vi "beginOneTouchShot.vi"(4 "Gap Coord":dbl[](array[numeric]), 6 "bestY":dbl, 8 "error in (no error)":errorcluster, 9 "Robot":refnum<class "Robot.lvclass">, 10 "Game":refnum<class "Game.lvclass">, 11 "ShootTactic in":refnum<class "ShootTactic.lvclass">) -> (0 "error out":errorcluster, 2 "Boolean":bool, 3 "ShootTactic out":refnum<class "ShootTactic.lvclass">)   [LabVIEW 2023]
uses:
  ShootTactic.lvclass
  Game_class/Game.lvclass
  Robot_class/Robot.lvclass
  Game_class/Game.lvclass/Game.ctl
  Robot_class/Robot.lvclass/Robot.ctl
  Parameters_class/Parameters.lvclass/Parameters.ctl
  Parameters_class/Read AttakingOurselves.vi
  Robot_class/Read role.vi
  Robot_class/Read Zone.vi
  Game_class/Read Parameters.lvclass.vi
  Game_class/Read BallRef.vi
  Game_class/Read KeeperTeam.vi
  Game_class/Read NewParameters.vi
  Game_class/Read FieldRef.vi
  Parameters_class/Parameters.lvclass
  Ball_class/Ball.lvclass
  Ally_class/Ally.lvclass
  Utilities_class/Style.ctl
  Field_class/Field.lvclass
  Zone_class/Zone.lvclass
  Team_class/KeeperPlay.ctl
  Utilities_class/Utilities.lvclass
panel:
  out "Evaluation":dbl
  out "appended array":bool[](array[boolean])
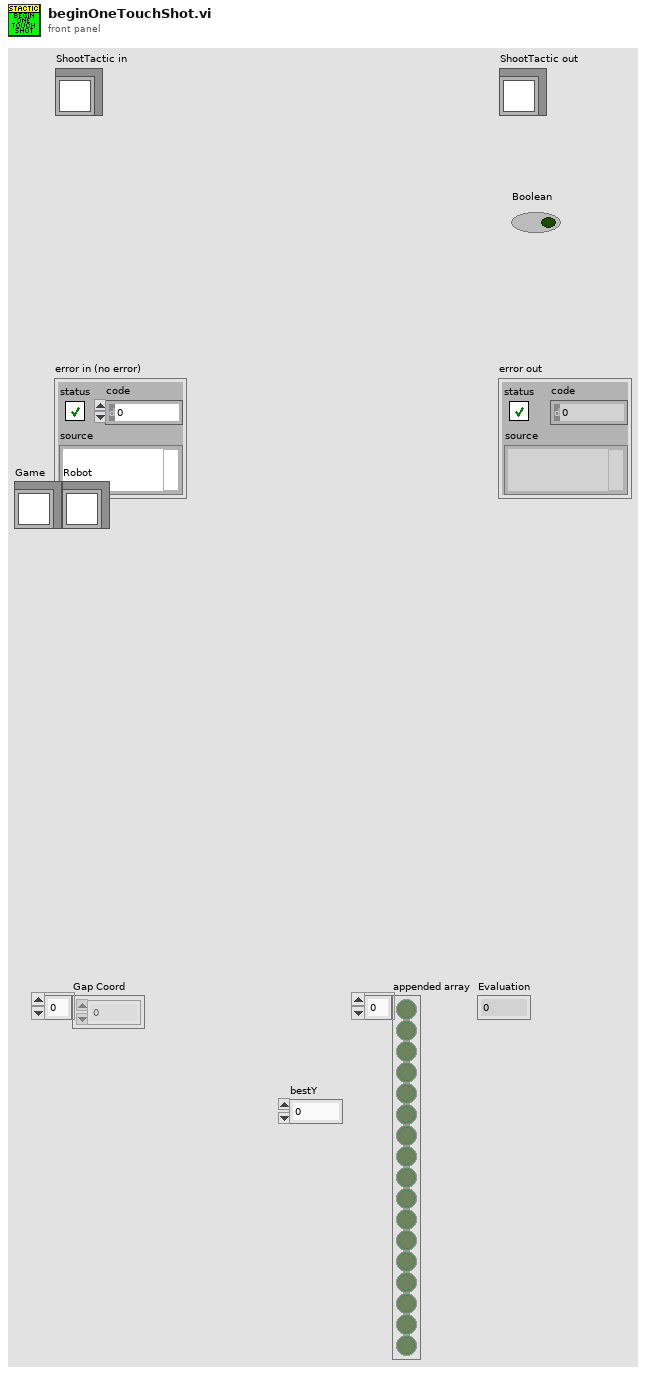
[diagram p1: front panel]
types:
  T1 = typedef "NewParameters.ctl" = cluster{"PenaltyDistance":dbl, "DistanceAttackerToBackBall":dbl, "Division":enum16{"Div B", "Div A"}, "DistanceToAvoidyEnemyRobot":dbl, "BallPlacementDistance":dbl, "DisatanceBehindBallToStealBall":dbl, "MaxDistanceToPositionKickoff":dbl, "BlockEnemyTarget":bool, "MaxStopVAng":dbl, "DistanceMarkerToEnemy":dbl, "IgnoreDribblerContact":bool, "DistanceToBeginEnemyPosession":dbl, "GoToBallWhenEnemyNotMoving":bool, "EnemyDistanceToReduceVelocity":dbl, "TurnOnEnemyDistanceToReduceVelocity":bool, "EnemyDistanceToShootOutBall":dbl, "DefenseKickBall":bool, "MoreKickToGoal? (0-0.3)":dbl, "ChipKickInEnemyField":bool, "ShootOutRobotId":dbl, "FieldLenghtDenominatorInShootOut":dbl, "AdjustPositionInBallPlacement":bool, "PowerGodPass":dbl, "VelocityAbortEnemyPos":dbl, "MaxDistToBeginPass":dbl, "MinDistToBeginPass":dbl, "VelocityInDirects":dbl, "BadDribblerIDs":i32[], "NewKickToDistanceAroundBall":dbl, "PowerAvoidColisionMarker":dbl, "DistanceToAvoidColisionMarker":dbl, "AvoidBallKick":dbl, "DistanceTryKick":dbl, "SuicideKickDIstance":dbl, "AdjustFirstKickDistance":dbl, "AvoidAimLessKick":dbl, "DistanceToAvoidyEnemyShootRobot ":dbl, "NumberOfMarkers":dbl, "PotField":bool, "PIDLateral":bool, "MinDistanceFirstKickX":dbl, "MinDistanceFirstKickY":dbl, "FractionOfDistToTouchGround\nAfterChipKick":dbl, "FractionOfKickxWhen\nComposedWithKickz":dbl, "Style":T2, "MoveInTurnState":bool, "DistFromEnemyToConsider\nMoveInTurnState":dbl, "CascadePID":bool, "TurnAroundParameters":cluster{"Radius":dbl, "Multiplier":dbl, "ChordAngle":dbl}, "SafeDriveVel":dbl, "DistanceToGoToBackBall":dbl, "minDistanceToNotFinish\nEnemyPossession":dbl, "OneTouchShot":cluster{"angleFactor":dbl, "maxAngle":dbl, "Attack":bool, "Defense":bool}, "OpenAngleToGoal":cluster{"minAngle":dbl, "maxAngle":dbl, "minEvaluation":dbl}, "ShotInterception":cluster{"shotSpeed":dbl, "minEnemySpeed":dbl, "maxEnemySpeed":dbl, "minEvaluation":dbl}, "AllyTeamArray":T3[], "maxDefendersNumber":i32, "Zone":cluster{"GuardPositionArray":dbl[][], "ZoneMidField":dbl[], "CenterForwardWidth":dbl}, "MinEvaluationToShoot":dbl, "PassInterception":cluster{"maxPassSpeed":dbl, "minPassSpeed":dbl, "minEnemySpeed":dbl, "chipPassDistance":dbl, "chipPassEvaluation":dbl, "minEvaluation":dbl, "maxEnemySpeed":dbl}, "PassDistance":cluster{"maxDistance":dbl, "minDistance":dbl}, "receiverSpeed":dbl, "maxBallSpeed":dbl, "slackTime":dbl, "Turning radius":dbl, "Turning v_ang":dbl, "AlignError":cluster{"Distance":dbl, "Orientation":dbl, "V_norm(m/s)":dbl, "V_ang (rad/s)":dbl}, "RobotRadius":dbl, "KickerDistance":dbl, "keeper angle  to cover goalpost":dbl}
  T2 = typedef "Style.ctl" = enum16{"Insanity", "Offensive", "Defensive"}
  T3 = typedef "AllyTeam.ctl" = enum16{"Keeper", "Defender", "Attacker"}
  T4 = typedef "KeeperPlay.ctl" = enum16{"SimpleBallPlacementAlly", "BallPlacementAlly", "BallPlacementEnemy", "ZigZag", "Goto", "NormalGame", "KeeperPlay", "Halt", "Timeout", "PenaltyEnemy", "TestPlay"}
  T5 = typedef "roles.ctl" = enum16{"SimpleBallPlacement", "BallPlacementAllyPasser", "BallPlacementAllyReceiver", "BallPlacementEnemy", "5Robots5th", "PassBestReceiver", "5Robots4th", "5Robots3rd", "5Robots2nd", "5Robots1st", "PassBestRobot", "WaitPass", "ABCThirdKicker", "ABCFirstKicker", "ABCSecondKicker", "Tabler", "TableFinalizer", "PrepareRollToPassRoller", "PrepareRollToPassReceiver", "SimplePassRoll", "SimplePassRollReceiver", "PenaltyDefense", "PreparePassReceiver 2", "PreparePassReceiver 1", "PassObserver", "Timeout", "Goto", "ZigZag", "None", "BallOutOfField", "DefenderArea", "Duelist", "AttackerStop", "FollowAttacker", "KeeperRole", "KickPenalty", "AttackerAimGoal", "AttackerBlock", "Marker", "Halt", "Shoot", "PassKicker", "PassReceiver", "TestRole", "PenaltyAttacker"}
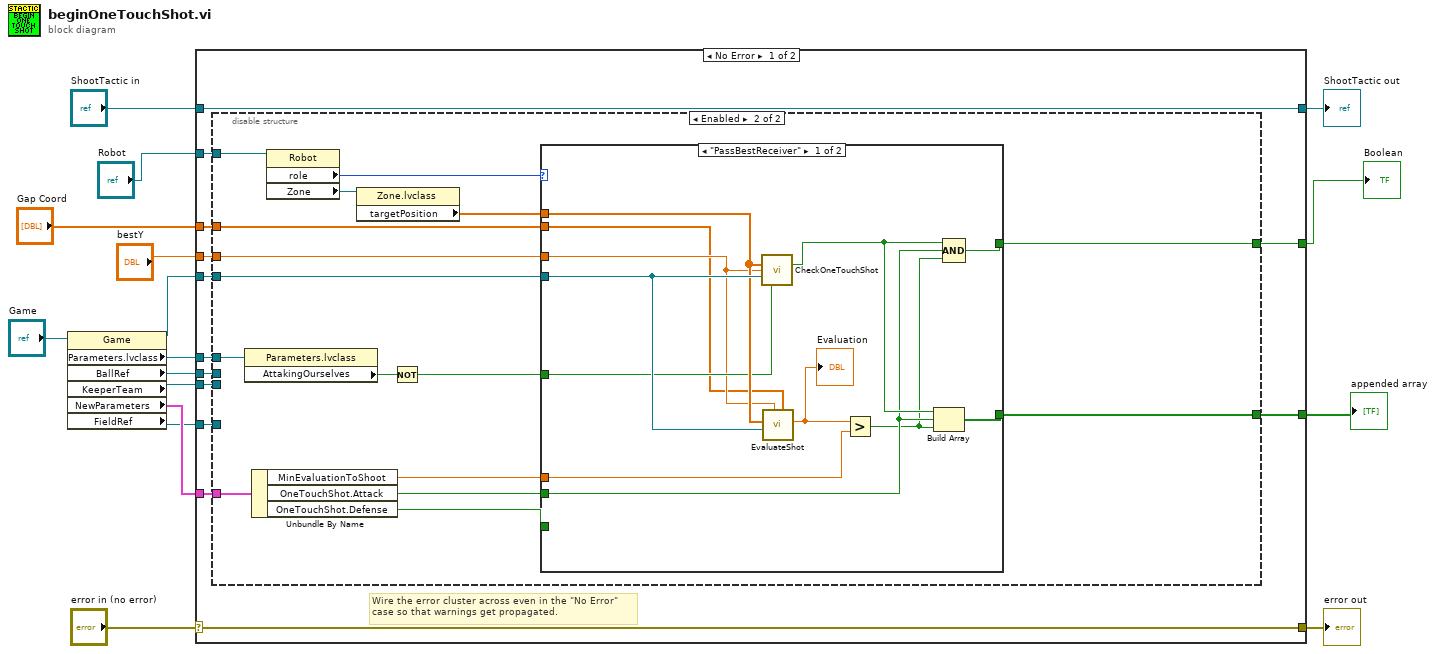
[diagram p0: block diagram]
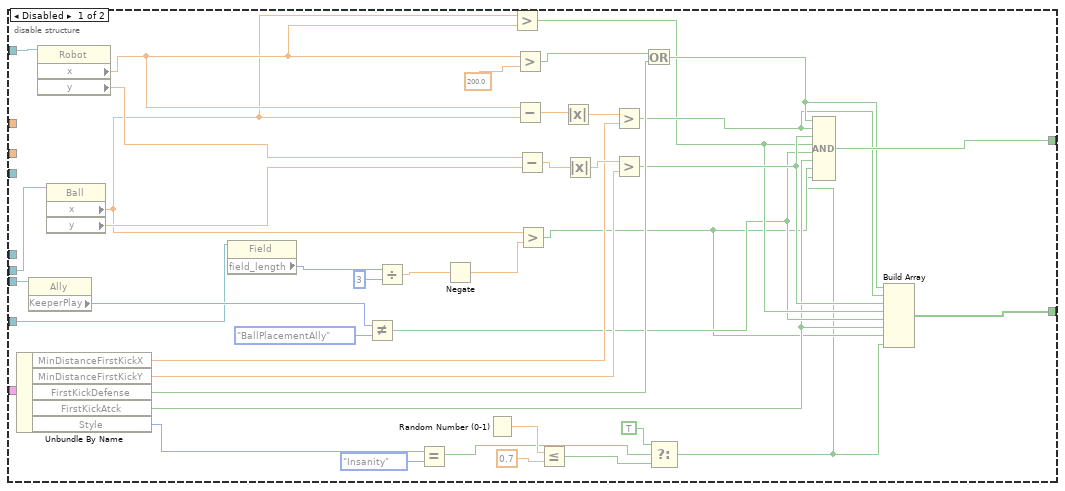
[diagram p2: hidden frame]
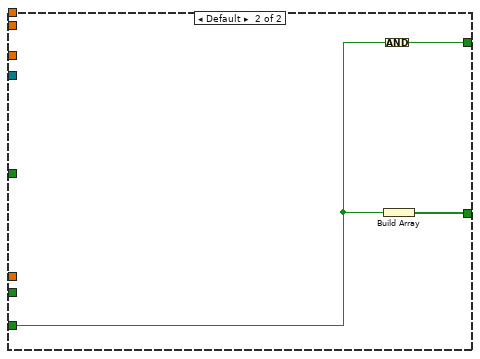
[diagram p3: hidden frame]
diagram:
  n1 = property class="Game"(reference="Game") -> (reference out=w6:refnum<class "Game.lvclass">, "Parameters.lvclass"=w2:refnum<class "Parameters.lvclass">, "BallRef"=w11:refnum<class "Ball.lvclass">, "KeeperTeam"=w12:refnum<class "Ally.lvclass">, "NewParameters"=w9:T1, "FieldRef"=w7:refnum<class "Field.lvclass">)  [unwired: 1 in, 1 out]
  n2 = case shown="No Error" "error in (no error)" {
    selector: "error in (no error)" -> [w28 w103]
    tunnel: [w28 w103] -> w15
    tunnel: [w29 w102] -> w13
    tunnel: "ShootTactic in" -> [w29 w102]
    tunnel: w12 -> [w27 _]
    tunnel: w11 -> [w26 _]
    tunnel: "Robot" -> [w25 _]
    tunnel: w9 -> [w18 _]
    tunnel: [w24 _] -> w5
    tunnel: [w23 _] -> w8
    tunnel: w7 -> [w22 _]
    tunnel: w6 -> [w21 _]
    tunnel: "bestY" -> [w20 _]
    tunnel: w2 -> [w19 _]
    tunnel: "Gap Coord" -> [w17 _]
    frame No Error {
      # "Wire the error cluster across even in the \"No Error\"\ncase so that warnings get propagated."
      n3 = disable-structure shown="Enabled" {
        disable-tunnel: w27 -> [w69 _]
        disable-tunnel: w26 -> [w67 _]
        disable-tunnel: w25 -> [w66 w86]
        disable-tunnel: w18 -> [w59 w84]
        disable-tunnel: [w55 w82] -> w24
        disable-tunnel: [w45 w83] -> w23
        disable-tunnel: w22 -> [w43 _]
        disable-tunnel: w21 -> [_ w81]
        disable-tunnel: w20 -> [_ w78]
        disable-tunnel: w19 -> [_ w76]
        disable-tunnel: w17 -> [_ w73]
        frame Disabled {
          n4 = Unbundle By Name(w59) -> ("MinDistanceFirstKickX"=w57:dbl, "MinDistanceFirstKickY"=w56:dbl, "FirstKickDefense"=w58:bool, "FirstKickAtck"=w46:bool, "Style"=w36:T2)
          n5 = property class="Ally"(reference=w69) -> ("KeeperPlay"=w68:T4)  [unwired: 1 in, 2 out]
          n6 = property class="Robot"(reference=w66) -> ("x"=w54:dbl, "y"=w52:dbl)  [unwired: 1 in, 2 out]
          n7 = property class="Ball"(reference=w67) -> ("x"=w44:dbl, "y"=w53:dbl)  [unwired: 1 in, 2 out]
          n8 = property class="Field"(reference=w43) -> ("field_length"=w42:i32)  [unwired: 1 in, 2 out]
          n9 = Not Equal?(x=w68, y=KeeperPlay."BallPlacementAlly") -> (x != y?=w47:bool)
          n10 = Divide(x=w42, y=3) -> (x/y=w40:dbl)
          n11 = Equal?(x=w36, y=Style."Insanity") -> (x = y?=w33:bool)
          n12 = Negate(x=w40) -> (-x=w39:dbl)
          n13 = Random Number (0-1)() -> (number: 0 to 1=w38:dbl)
          n14 = Greater?(x=w44, y=w54) -> (0:w48:bool)
          n15 = Greater?(x=w54, y=200.0) -> (0:w60:bool)
          n16 = Subtract(x=w54, y=w44) -> (x-y=w64:dbl)
          n17 = Subtract(x=w52, y=w53) -> (x-y=w63:dbl)
          n18 = Greater?(x=w44, y=w39) -> (0:w31:bool)
          n19 = Less Or Equal?(x=w38, y=0.7) -> (x <= y?=w34:bool)
          n20 = Absolute Value(x=w64) -> (abs(x)=w62:dbl)
          n21 = Absolute Value(x=w63) -> (abs(x)=w61:dbl)
          n22 = Greater?(x=w62, y=w57) -> (0:w50:bool)
          n23 = Greater?(x=w61, y=w56) -> (0:w49:bool)
          n24 = Or(x=w60, y=w58) -> (x .or. y?=w51:bool)
          n25 = Select(t=TRUE, s=w33, f=w34) -> (s? t:f=w30:bool)
          n26 = Compound Arithmetic op=AND(w51, w50, w49, w48, w47, w46, w31, w30) -> (w55:bool)
          n27 = Build Array(w51, w50, w49, w48, w47, w46, w31, w30) -> (w45:bool[])
        }
        frame Enabled {
          n28 = property class="Parameters.lvclass"(reference=w76) -> ("AttakingOurselves"=w75:bool)  [unwired: 1 in, 2 out]
          n29 = Unbundle By Name(w84) -> ("MinEvaluationToShoot"=w77:dbl, "OneTouchShot.Attack"=w79:bool, "OneTouchShot.Defense"=w80:bool)
          n30 = property class="Robot"(reference=w86) -> ("role"=w85:T5, "Zone"=w72:refnum<class "Zone.lvclass">)  [unwired: 1 in, 2 out]
          n31 = property class="Zone.lvclass"(reference=w72) -> ("targetPosition"=w71:dbl[])  [unwired: 1 in, 2 out]
          n32 = Not(x=w75) -> (.not. x?=w74:bool)
          n33 = case shown="\"PassBestReceiver\"" w85 {
            tunnel: [w96 w101] -> w83
            tunnel: [w98 w100] -> w82
            tunnel: w81 -> [w91 _]
            tunnel: w71 -> [w90 _]
            tunnel: w80 -> [_ w99]
            tunnel: w79 -> [w95 _]
            tunnel: w77 -> [w93 _]
            tunnel: w78 -> [w88 _]
            tunnel: w74 -> [w89 _]
            tunnel: w73 -> [w87 _]
            frame "PassBestReceiver" {
              n34 = call "CheckOneTouchShot.vi"("Point"=w90, "Best y"=w88, "Game"=w91, "Ally?"=w89) -> ("OneTouch"=w97:bool)  [unwired: 8 in, 3 out]
              n35 = call "EvaluateShot.vi"("Gap Coord"=w87, "BestY"=w88, "Game"=w91, "Point"=w90) -> ("Evaluation"=w92:dbl)  [unwired: 5 in, 2 out]
              "Evaluation" <- w92
              n36 = Greater?(x=w92, y=w93) -> (0:w94:bool)
              n37 = Build Array(w97, w95, w94) -> (w96:bool[])
              n38 = Compound Arithmetic op=AND(w97, w95, w94) -> (w98:bool)
            }
            frame Default {
              n39 = Build Array(w99) -> (w101:bool[])
              n40 = Compound Arithmetic op=AND(w99) -> (w100:bool)
            }
          }
        }
      }
    }
    frame Error {
    }
  }
  "error out" <- w15
  "ShootTactic out" <- w13
  "Boolean" <- w5
  "appended array" <- w8
